vi "Control - Generic - Low-Idle Governor Host.vi"() -> ()   [LabVIEW 2015, in "ECS-Host.lvlib"]
uses:
  ECS-Host.lvlib
  <vilib>/addons/Software Calibration Management/XControls/TBL1D.xctl
panel:
  out "PedalOut":sgl caption="[]"
  out "PedalIn":sgl caption="[%]"
  out "LIG_DEffort":sgl caption="[]"
  out "LIG_IEffort":sgl caption="[]"
  out "LIG_PEffort":sgl caption="[]"
  in  "LIG_IntMin":sgl caption="[]"
  in  "LIG_IntMax":sgl caption="[]"
  in  "LIG_DerMin":sgl caption="[]"
  in  "LIG_DerMax":sgl caption="[]"
  out "LIG_PIDOut":sgl caption="[]"
  in  "LIG_Kd":sgl caption="[]"
  in  "LIG_PIDMin":sgl caption="[]"
  in  "LIG_PIDMax":sgl caption="[]"
  in  "LIG_Ki":sgl caption="[%-sec/RPM]"
  in  "LIG_Kp":sgl caption="[%/RPM]"
  in  "IdleSpeed_ManE":bool
  in  "IdleSpeed_Man":sgl caption="[RPM]"
  out "IdleSpeed_TblOut":sgl caption="[RPM]"
  in  "LIG_E":bool
  in  "IdleSpeed_Tbl":cluster{"X":sgl[], "Y":sgl[]}(xcontrol)
  # "[C]"
  # "[RPM]"
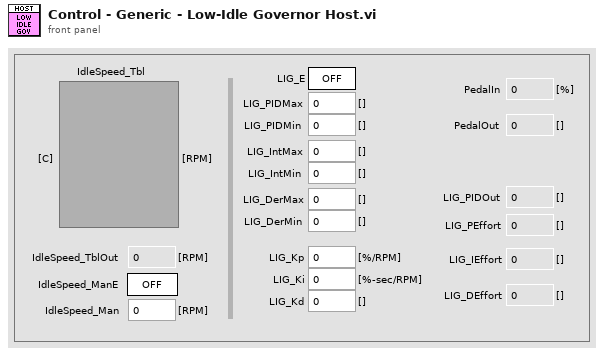
[diagram p1: front panel]
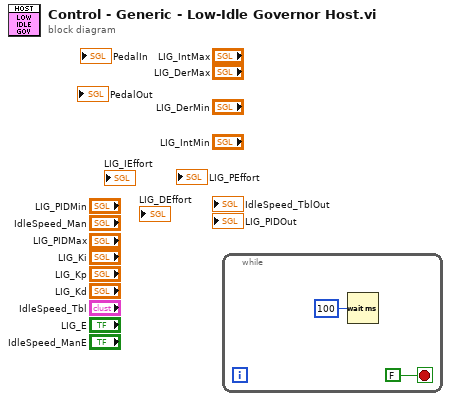
[diagram p0: block diagram]
diagram:
  n1 = while {
    stop <- FALSE stop-if-true
    n2 = Wait (ms)(milliseconds to wait=u32 100) -> ()  [unwired: 1 out]
  }
